vi "get_plot-command_and_remove.vi"(8 "error in (no error)":errorcluster, 11 "Plots in":refnum<class "Plots.lvclass">) -> (0 "error out":errorcluster, 1 "new command?":bool, 2 "plot command out":string, 3 "Plots out":refnum<class "Plots.lvclass">, 4 "variant data":variant)   [LabVIEW 2018, in "Plots.lvclass"]
doc: "reads the private property \"plot-command\" and sets it to an empty string thus removes the command from the property.\nThe command is split into the actual command string and the parameters"
uses:
  Plots.lvclass
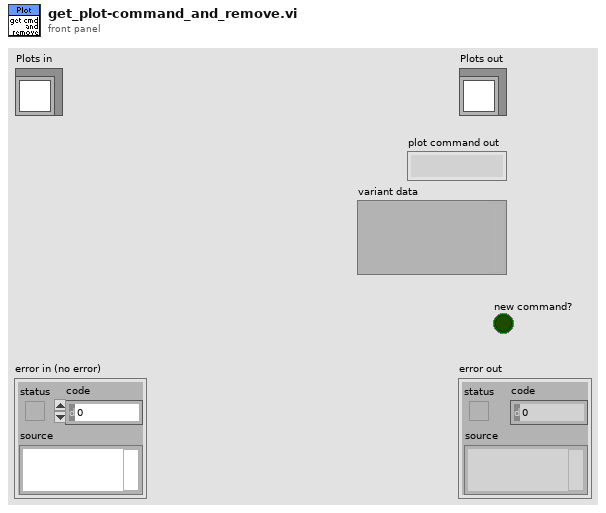
[diagram p1: front panel]
types:
  T1 = cluster{"command":string, "variant data":variant}
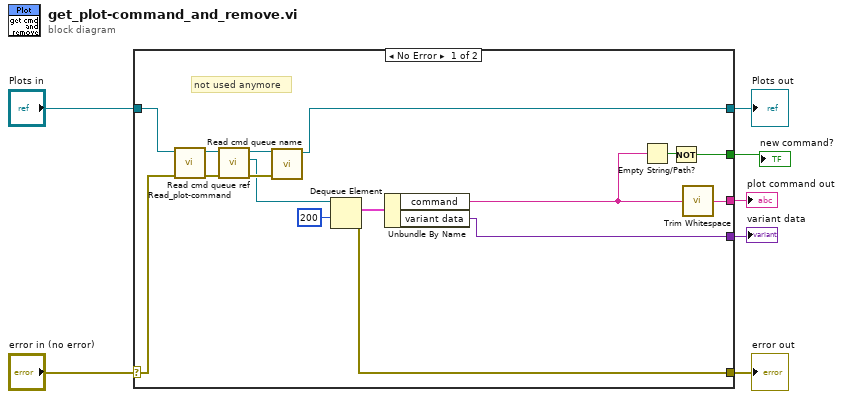
[diagram p0: block diagram]
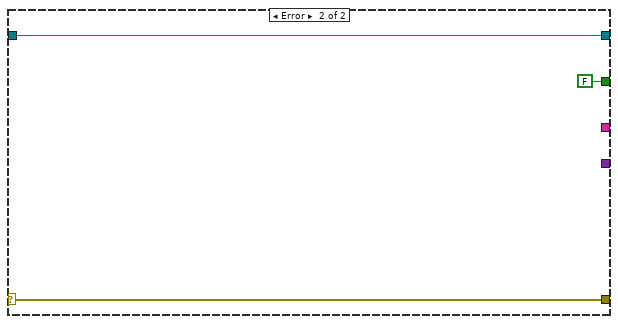
[diagram p2: hidden frame]
diagram:
  n1 = case shown="No Error" "error in (no error)" {
    selector: "error in (no error)" -> [w22 w26]
    tunnel: [w17 w26] -> w6
    tunnel: [w14 w25] -> w4
    tunnel: "Plots in" -> [w23 w25]
    tunnel: [w21 _] -> w3
    tunnel: [w11 _] -> w2
    tunnel: [w8 FALSE] -> w1
    frame No Error {
      # "not used anymore"
      n2 = call-dynamic "Read_plot-command.vi"("error in (no error)"=w22, "Plots in"=w23) -> ("error out"=w19:errorcluster, "Plots out"=w20:refnum<class "Plots.lvclass">)  [unwired: 7 in, 1 out]
      n3 = call-dynamic "Read cmd queue ref.vi"("error in (no error)"=w19, "Plots in"=w20) -> ("error out"=w15:errorcluster, "cmd queue"=w13:refnum<queue>, "Plots out"=w16:refnum<class "Plots.lvclass">)  [unwired: 7 in]
      n4 = call-dynamic "Read cmd queue name.vi"("error in (no error)"=w15, "Plots in"=w16) -> ("Plots out"=w14:refnum<class "Plots.lvclass">)  [unwired: 7 in, 2 out]
      n5 = Dequeue Element(queue=w13, timeout in ms (-1)=200) -> (element=w12:T1, error out=w17:errorcluster)  [unwired: 1 in, 2 out]
      n6 = Unbundle By Name(w12) -> ("command"=w10:string, "variant data"=w11:variant)
      n7 = Empty String/Path?(string/path=w10) -> (empty?=w9:bool)
      n8 = Not(x=w9) -> (.not. x?=w8:bool)
      n9 = call <vilib>:"Trim Whitespace.vi"("string"=w10) -> ("trimmed string"=w21:string)  [unwired: 1 in]
    }
    frame Error {
    }
  }
  "error out" <- w6
  "Plots out" <- w4
  "plot command out" <- w3
  "variant data" <- w2
  "new command?" <- w1
